vi "Inclinometer.vi"   [LabVIEW 2016]
uses:
  ModbusCRC/CRC16Settings.ctl
types:
  T1 = typedef "CRC16Settings.ctl" = cluster{"DataFIFO":refnum<k21>, "CalculateFIFO":refnum<k21>, "CRCFIFO":refnum<k21>}
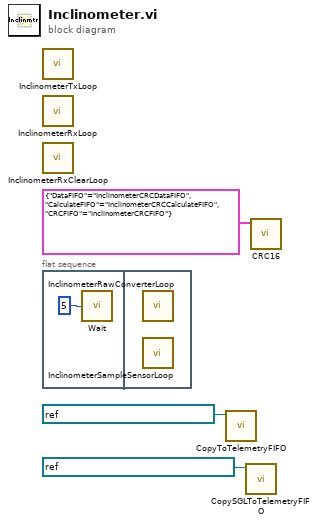
[diagram p0: block diagram]
diagram:
  n1 = call "InclinometerTxLoop.vi"() -> ()  [unwired: 12 in]
  n2 = call "InclinometerRxLoop.vi"() -> ()  [unwired: 12 in]
  n3 = call "InclinometerRxClearLoop.vi"() -> ()  [unwired: 12 in]
  n4 = flat-sequence {
    frame #0 {
      n5 = call "Wait"("Count(mSec)"=u32 5) -> ()  [unwired: 1 out]
    }
    frame #1 {
      n6 = call "InclinometerRawConverterLoop.vi"() -> ()  [unwired: 12 in]
      n7 = call "InclinometerSampleSensorLoop.vi"() -> ()  [unwired: 12 in]
    }
  }
  n8 = call "CopyToTelemetryFIFO.vi"("SourceFIFO"=refnum<k21> "InclinometerTelemetryFIFO") -> ()  [unwired: 11 in]
  n9 = call "CopySGLToTelemetryFIFO.vi"("SourceFIFO"=refnum<k21> "InclinometerTelemetrySGLFIFO") -> ()  [unwired: 11 in]
  n10 = call "CRC16.vi"("CRC16Settings"=T1 {"DataFIFO"="InclinometerCRCDataFIFO", "CalculateFIFO"="InclinometerCRCCalculateFIFO", "CRCFIFO"="InclinometerCRCFIFO"} ("ModbusCRCSettings")) -> ()  [unwired: 11 in]
